vi "XY Sine Graph Express.vi"() -> ()   [LabVIEW 2020]
panel:
  in  "stop":bool
  out "XY Graph":cluster{"Y":dbl[], "Y":dbl[]}[](graph)
  in  "Phase":dbl(knob) scale=0.0..180.0
  in  "Phase":dbl(knob) scale=0.0..180.0
  in  "Frequency":dbl(knob) scale=0.0..200.0
  in  "Frequency":dbl(knob) scale=0.0..200.0
  in  "Amplitude":dbl(knob) scale=0.0..10.0
  in  "Amplitude":dbl(knob) scale=0.0..10.0
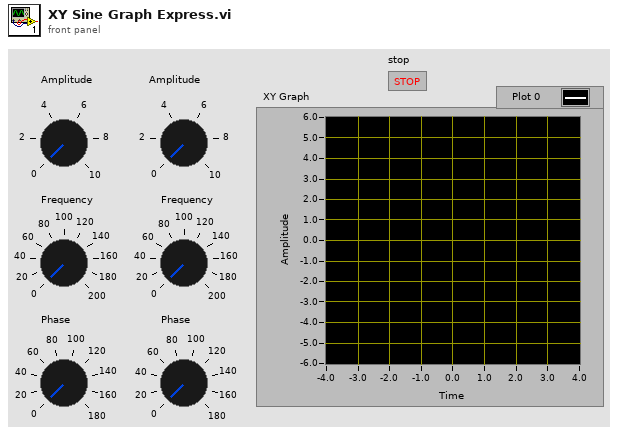
[diagram p1: front panel]
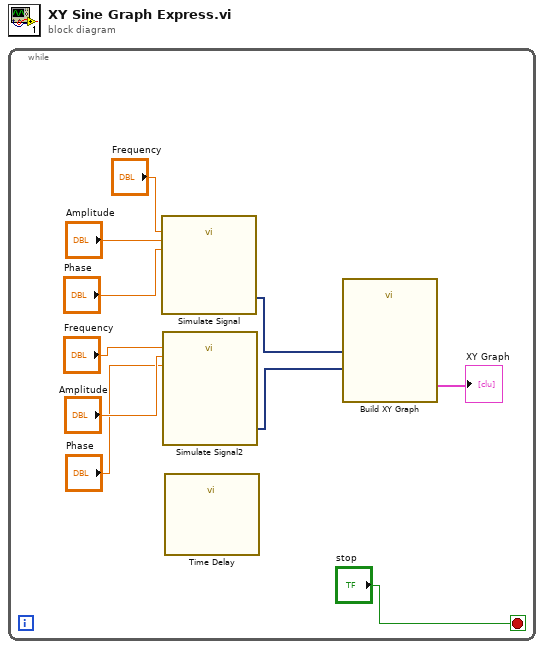
[diagram p0: block diagram]
diagram:
  n1 = while {
    stop <- "stop" stop-if-true
    n2 = call "Simulate Signal"("Frequency"="Frequency", "Amplitude"="Amplitude", "Phase"="Phase") -> ("Sine"=w10:dynamicdata)  [unwired: 11 in, 1 out]
    n3 = call "Simulate Signal2"("Frequency"="Frequency", "Amplitude"="Amplitude", "Phase"="Phase") -> ("Sine"=w9:dynamicdata)  [unwired: 11 in, 1 out]
    n4 = call "Time Delay"() -> ()  [unwired: 11 in, 1 out]
    n5 = call "Build XY Graph"("Y Input"=w9, "X Input"=w10) -> ("XY Graph"=→"XY Graph":cluster{"X":dbl[], "Y":dbl[]}[])  [unwired: 8 in, 1 out]
  }
